vi "count_clients_recursively_VCTP.vi"(7 "Nested type desc.":cluster{"Type descriptor":u8, "Data":string} {"Type descriptor" items=["Void"=0, "NumberI8"=1, "NumberI16"=2, "NumberI32"=3, "NumberI64"=4, "NumberU8"=5, "NumberU16"=6, "NumberU32"=7, "NumberU64"=8, "NumberSGL"=9, "NumberDBL"=10, "NumberEXT"=11, "NumberCSG"=12, "NumberCDB"=13, "NumberCXT"=14, "UnitI8"=17, "UnitI16"=18, "UnitI32"=19, "UnitI64"=20, "UnitU8"=21, "UnitU16"=22, "UnitU32"=23, "UnitU64"=24, "UnitSGL"=25, "UnitDBL"=26, "UnitEXT"=27, "UnitCSG"=28, "UnitCDB"=29, "UnitCXT"=30, "BoolU16"=32, "Bool"=33, "String"=48, "String2"=49, "Path"=50, "Picture"=51, "CString"=52, "PascalString"=53, "Tag"=55, "SubString"=63, "Array"=64, "ArrayDataPtr"=65, "SubArray"=79, "Cluster"=80, "LVVariant"=83, "MeasureData"=84, "ComplexFixedPt"=94, "FixedPoint"=95, "Block"=96, "TypeBlock"=97, "VoidBlock"=98, "AlignedBlock"=99, "RepeatedBlock"=100, "AlignmntMarker"=101, "Refnum"=112, "Set"=115, "Map"=116, "PointerNumber"=128, "PointerNumberI8"=129, "PointerNumberI16"=130, "PointerNumberI32"=131, "PointerNumberI64"=132, "PointerNumberU8"=133, "PointerNumberU16"=134, "PointerNumberU32"=135, "PointerNumberU64"=136, "PointerNumberSGL"=137, "PointerNumberDBL"=138, "PointerNumberEXT"=139, "PointerNumberCSG"=140, "PointerNumberCDB"=141, "PointerNumberCXT"=142, "ArrayInterfc"=160, "InterfcToData"=161, "Terminal"=240, "TypeDef"=241, "PolyVI"=242]}, 8 "error in (no error)":errorcluster, 9 "Control counts in (0)":T1, 10 "Type descriptor index":i32, 11 "VCTP type descriptor list":refnum<data-value>) -> (0 "error out":errorcluster, 1 "Control counts out":T1, 3 "Type descriptor list dup":refnum<data-value>)   [LabVIEW 2020]
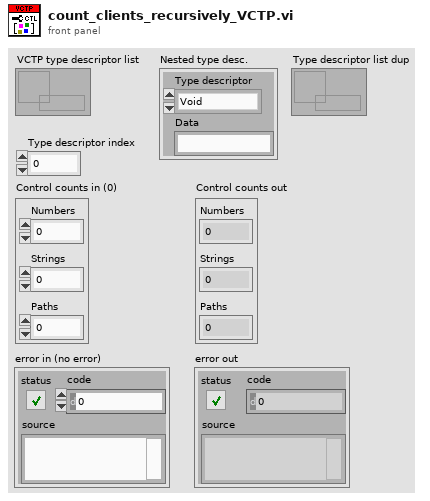
[diagram p1: front panel]
types:
  T1 = cluster{"Numbers":i32, "Strings":i32, "Paths":i32}
  T2 = cluster{"field0":i16, "field2":i16, "field4":i16, "idx":i16}[]
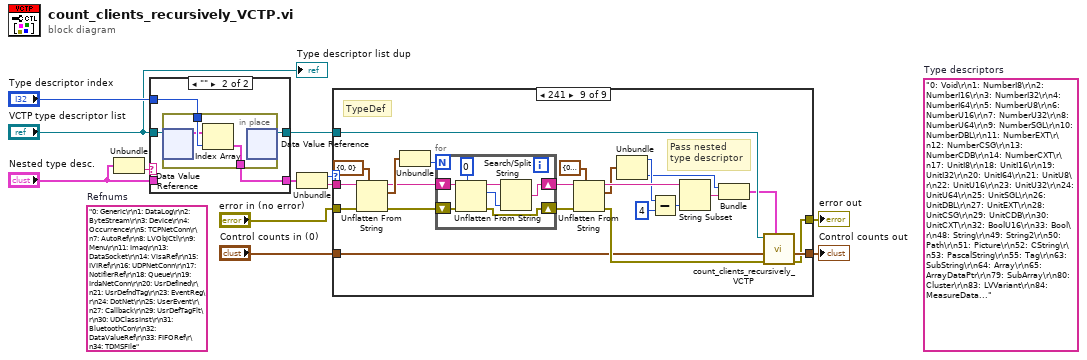
[diagram p0: block diagram]
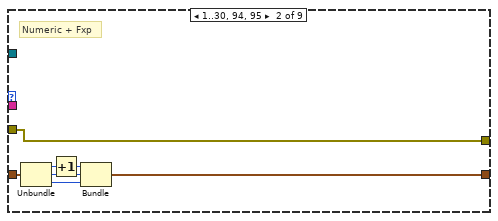
[diagram p4: hidden frame]
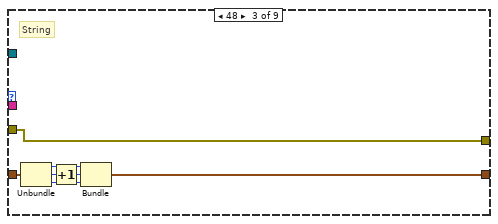
[diagram p5: hidden frame]
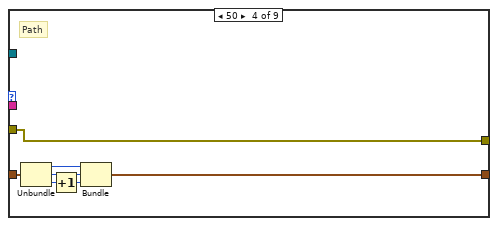
[diagram p6: hidden frame]
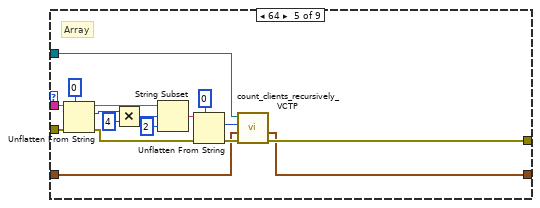
[diagram p7: hidden frame]
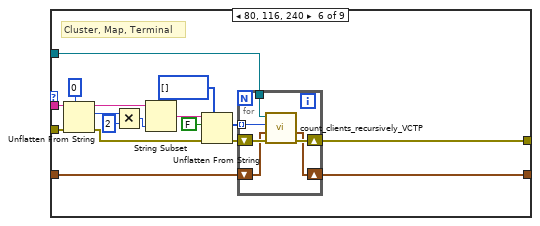
[diagram p8: hidden frame]
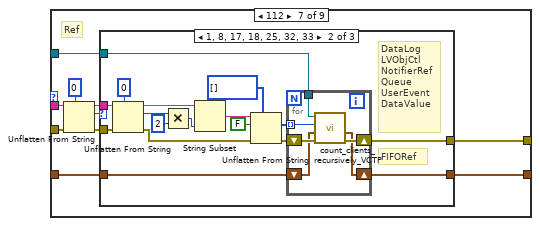
[diagram p9: hidden frame]
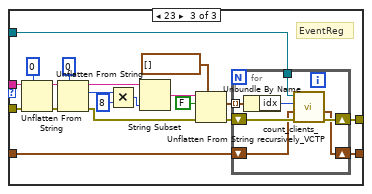
[diagram p11: hidden frame]
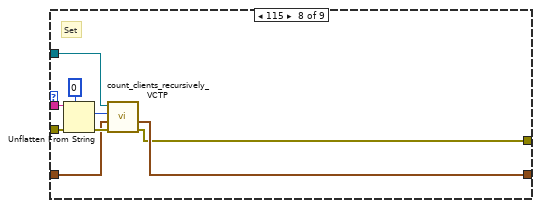
[diagram p12: hidden frame]
diagram:
  (unwired) "0: Generic\r\n1: DataLog\r\n2: ByteStream\r\n3: Device\r\n4: Occurrence\r\n5: TCPNetConn\r\n7: AutoRef\r\n8: LVObjCtl\r\n9: Menu\r\n11: Imaq\r\n13: DataSocket\r\n14: VisaRef\r\n15: IVIRef\r\n16: UDPNetConn\r\n17: NotifierRef\r\n18: Queue\r\n19: IrdaNetConn\r\n20: UsrDefined\r\n21: UsrDefndTag\r\n23: EventReg\r\n24: DotNet\r\n25: UserEvent\r\n27: Callback\r\n29: UsrDefTagFlt\r\n30: UDClassInst\r\n31: BluetoothCon\r\n32: DataValueRef\r\n33: FIFORef\r\n34: TDMSFile"  # Refnums
  (unwired) "0: Void\r\n1: NumberI8\r\n2: NumberI16\r\n3: NumberI32\r\n4: NumberI64\r\n5: NumberU8\r\n6: NumberU16\r\n7: NumberU32\r\n8: NumberU64\r\n9: NumberSGL\r\n10: NumberDBL\r\n11: NumberEXT\r\n12: NumberCSG\r\n13: NumberCDB\r\n14: NumberCXT\r\n17: UnitI8\r\n18: UnitI16\r\n19: UnitI32\r\n20: UnitI64\r\n21: UnitU8\r\n22: UnitU16\r\n23: UnitU32\r\n24: UnitU64\r\n25: UnitSGL\r\n26: UnitDBL\r\n27: UnitEXT\r\n28: UnitCSG\r\n29: UnitCDB\r\n30: UnitCXT\r\n32: BoolU16\r\n33: Bool\r\n48: String\r\n49: String2\r\n50: Path\r\n51: Picture\r\n52: CString\r\n53: PascalString\r\n55: Tag\r\n63: SubString\r\n64: Array\r\n65: ArrayDataPtr\r\n79: SubArray\r\n80: Cluster\r\n83: LVVariant\r\n84: MeasureData\r\n94: ComplexFixedPt\r\n95: FixedPoint\r\n96: Block\r\n97: TypeBlock\r\n98: VoidBlock\r\n99: AlignedBlock\r\n100: RepeatedBlock\r\n101: AlignmntMarker\r\n112: Refnum\r\n115: Set\r\n116: Map\r\n128: PointerNumber\r\n129: PointerNumberI8\r\n130: PointerNumberI16\r\n131: PointerNumberI32\r\n132: PointerNumberI64\r\n133: PointerNumberU8\r\n134: PointerNumberU16\r\n135: PointerNumberU32\r\n136: PointerNumberU64\r\n137: PointerNumberSGL\r\n138: PointerNumberDBL\r\n139: PointerNumberEXT\r\n140: PointerNumberCSG\r\n141: PointerNumberCDB\r\n142: PointerNumberCXT\r\n160: ArrayInterfc\r\n161: InterfcToData\r\n240: Terminal\r\n241: TypeDef\r\n242: PolyVI"  # Type descriptors
  n1 = Unbundle("Nested type desc.") -> ("Data"=w3:string)  [unwired: 1 out]
  n2 = case shown="\"\"" w3 {
    tunnel: "VCTP type descriptor list" -> [w14 w18]
    tunnel: "Type descriptor index" -> [_ w17]
    tunnel: [w13 w16] -> w11
    tunnel: [w14 w15] -> w6
    tunnel: "Nested type desc." -> [w13 _]
    frame Default {
    }
    frame "" {
      n3 = in-place {
        in-place-border: w17 -> [w21]
        in-place-border: [w19] -> w16
        n4 = in-place-dvr #1(w18) -> (w20:cluster{"Type descriptor":u8, "Data":string}[])  [unwired: 1 out]
        n5 = Index Array(array=w20, index=w21) -> (element=w19:cluster{"Type descriptor":u8, "Data":string})
        n6 = in-place-dvr #1() -> (w15:refnum<data-value>)  [unwired: 1 in, 1 out]
      }
    }
  }
  n7 = Unbundle(w11) -> ("Type descriptor"=w10:u8, "Data"=w8:string)
  n8 = case shown="241" w10 {
    tunnel: "error in (no error)" -> [w22 w24 w31 w38 w57 w66 w92 w153 w165]
    tunnel: [w23 w25 w35 w43 w45 w62 w86 w148 w159] -> w5
    tunnel: [w22 w24 w31 w38 w46 w63 w85 w147 w158] -> w4
    tunnel: "Control counts in (0)" -> [w23 w30 w37 w44 w47 w65 w87 w149 w160]
    tunnel: w8 -> [_ _ _ _ w58 w67 w94 w155 w164]
    tunnel: w6 -> [_ _ _ _ w50 w64 w88 w152 w157]
    frame Default {
    }
    frame 1..30, 94, 95 {
      # "Numeric + Fxp"
      n9 = Unbundle(w30) -> ("Numbers"=w29:i32, "Strings"=w27:i32, "Paths"=w26:i32)
      n10 = Increment(x=w29) -> (x+1=w28:i32)
      n11 = Bundle(w28, "Strings"=w27, "Paths"=w26) -> (w25:cluster{i32, "Strings":i32, "Paths":i32})  [unwired: 1 in]
    }
    frame 48 {
      # "String"
      n12 = Unbundle(w37) -> ("Numbers"=w34:i32, "Strings"=w33:i32, "Paths"=w36:i32)
      n13 = Increment(x=w33) -> (x+1=w32:i32)
      n14 = Bundle("Numbers"=w34, w32, "Paths"=w36) -> (w35:cluster{"Numbers":i32, i32, "Paths":i32})  [unwired: 1 in]
    }
    frame 50 {
      # "Path"
      n15 = Unbundle(w44) -> ("Numbers"=w42:i32, "Strings"=w40:i32, "Paths"=w41:i32)
      n16 = Increment(x=w41) -> (x+1=w39:i32)
      n17 = Bundle("Numbers"=w42, "Strings"=w40, w39) -> (w43:cluster{"Numbers":i32, "Strings":i32, i32})  [unwired: 1 in]
    }
    frame 64 {
      # "Array"
      n18 = Unflatten From String(type=i16 0, binary string=w58, error in (no error)=w57) -> (rest of the binary string=w56:string, value=w60:i16, error out=w51:errorcluster)  [unwired: 2 in]
      n19 = Multiply(x=w60, y=i16 4) -> (x*y=w55:i16)
      n20 = String Subset(string=w56, offset (0)=w55, length (rest)=2 ("length (rest)")) -> (substring=w52:string)
      n21 = Unflatten From String(type=i16 0, binary string=w52, error in (no error)=w51) -> (value=w49:i16, error out=w48:errorcluster)  [unwired: 2 in, 1 out]
      n22 = call "count_clients_recursively_VCTP.vi"("error in (no error)"=w48, "Control counts in (0)"=w47, "Type descriptor index"=w49, "VCTP type descriptor list"=w50) -> ("error out"=w46:errorcluster, "Control counts out"=w45:T1)  [unwired: 5 in, 1 out]
    }
    frame 80, 116, 240 {
      # "Cluster, Map, Terminal"
      n23 = Unflatten From String(type=i16 0, binary string=w67, error in (no error)=w66) -> (rest of the binary string=w76:string, value=w71:i16, error out=w72:errorcluster)  [unwired: 2 in]
      n24 = Multiply(x=w71, y=i16 2) -> (x*y=w77:i16)
      n25 = String Subset(string=w76, length (rest)=w77) -> (substring=w78:string)  [unwired: 1 in]
      n26 = Unflatten From String(type=i16[] [] ("index"), binary string=w78, data includes array or string size? (T)=FALSE, error in (no error)=w72) -> (value=w74:i16[], error out=w75:errorcluster)  [unwired: 1 in, 1 out]
      n27 = for {
        tunnel: w74 -> [w83] mode=indexing
        tunnel: w64 -> [w84]
        shift-right: [w81] -> w63
        shift-left: w75 -> [w82]
        shift-right: [w79] -> w62
        shift-left: w65 -> [w80]
        n28 = call "count_clients_recursively_VCTP.vi"("error in (no error)"=w82, "Control counts in (0)"=w80, "Type descriptor index"=w83, "VCTP type descriptor list"=w84) -> ("error out"=w81:errorcluster, "Control counts out"=w79:T1)  [unwired: 5 in, 1 out]
      }
    }
    frame 112 {
      # "Ref"
      n29 = Unflatten From String(type=i16 0, binary string=w94, error in (no error)=w92) -> (rest of the binary string=w91:string, value=w90:i16, error out=w89:errorcluster)  [unwired: 2 in]
      n30 = case shown="1, 8, 17, 18, 25, 32, 33" w90 {
        tunnel: w91 -> [_ w112 w124]
        tunnel: w89 -> [w96 w111 w123]
        tunnel: w88 -> [_ w104 w133]
        tunnel: w87 -> [w95 w102 w131]
        tunnel: [w95 w101 w130] -> w86
        tunnel: [w96 w100 w129] -> w85
        frame Default {
        }
        frame 1, 8, 17, 18, 25, 32, 33 {
          # "FIFORef"
          # "DataLog\nLVObjCtl\nNotifierRef\nQueue\nUserEvent\nDataValue"
          n31 = Unflatten From String(type=i16 0, binary string=w112, error in (no error)=w111) -> (rest of the binary string=w99:string, value=w108:i16, error out=w107:errorcluster)  [unwired: 2 in]
          n32 = Multiply(x=w108, y=i16 2) -> (x*y=w98:i16)
          n33 = String Subset(string=w99, length (rest)=w98) -> (substring=w97:string)  [unwired: 1 in]
          n34 = Unflatten From String(type=i16[] [] ("index"), binary string=w97, data includes array or string size? (T)=FALSE, error in (no error)=w107) -> (value=w105:i16[], error out=w103:errorcluster)  [unwired: 1 in, 1 out]
          n35 = for {
            tunnel: w105 -> [w118] mode=indexing
            tunnel: w104 -> [w119]
            shift-right: [w116] -> w100
            shift-left: w103 -> [w117]
            shift-right: [w114] -> w101
            shift-left: w102 -> [w115]
            n36 = call "count_clients_recursively_VCTP.vi"("error in (no error)"=w117, "Control counts in (0)"=w115, "Type descriptor index"=w118, "VCTP type descriptor list"=w119) -> ("error out"=w116:errorcluster, "Control counts out"=w114:T1)  [unwired: 5 in, 1 out]
          }
        }
        frame 23 {
          # "EventReg"
          n37 = Unflatten From String(type=i16 0, binary string=w124, error in (no error)=w123) -> (rest of the binary string=w122:string, error out=w121:errorcluster)  [unwired: 2 in, 1 out]
          n38 = Unflatten From String(type=i16 0, binary string=w122, error in (no error)=w121) -> (rest of the binary string=w128:string, value=w136:i16, error out=w135:errorcluster)  [unwired: 2 in]
          n39 = Multiply(x=w136, y=i16 8) -> (x*y=w127:i16)
          n40 = String Subset(string=w128, length (rest)=w127) -> (substring=w126:string)  [unwired: 1 in]
          n41 = Unflatten From String(type=T2 [], binary string=w126, data includes array or string size? (T)=FALSE, error in (no error)=w135) -> (value=w134:T2, error out=w132:errorcluster)  [unwired: 1 in, 1 out]
          n42 = for {
            tunnel: w134 -> [w141] mode=indexing
            tunnel: w133 -> [w146]
            shift-right: [w144] -> w129
            shift-left: w132 -> [w145]
            shift-right: [w142] -> w130
            shift-left: w131 -> [w143]
            n43 = Unbundle By Name(w141) -> ("idx"=w140:i16)
            n44 = call "count_clients_recursively_VCTP.vi"("error in (no error)"=w145, "Control counts in (0)"=w143, "Type descriptor index"=w140, "VCTP type descriptor list"=w146) -> ("error out"=w144:errorcluster, "Control counts out"=w142:T1)  [unwired: 5 in, 1 out]
          }
        }
      }
    }
    frame 115 {
      # "Set"
      n45 = Unflatten From String(type=i16 0, binary string=w155, error in (no error)=w153) -> (value=w151:i16, error out=w150:errorcluster)  [unwired: 2 in, 1 out]
      n46 = call "count_clients_recursively_VCTP.vi"("error in (no error)"=w150, "Control counts in (0)"=w149, "Type descriptor index"=w151, "VCTP type descriptor list"=w152) -> ("error out"=w147:errorcluster, "Control counts out"=w148:T1)  [unwired: 5 in, 1 out]
    }
    frame 241 {
      # "Pass nested\ntype descriptor"
      # "TypeDef"
      n47 = Unflatten From String(type=cluster{"Flags":i32, "NumStr":i32} {"Flags"=0, "NumStr"=0}, binary string=w164, error in (no error)=w165) -> (rest of the binary string=w166:string, value=w177:cluster{"Flags":i32, "NumStr":i32}, error out=w167:errorcluster)  [unwired: 2 in]
      n48 = Unbundle(w177) -> ("NumStr"=w178:i32)  [unwired: 1 out]
      n49 = for {
        N: w178 -> [_]
        shift-right: [w180] -> w171
        shift-left: w166 -> [w184]
        shift-right: [w179] -> w173
        shift-left: w167 -> [w183]
        n50 = Unflatten From String(type=u8 0, binary string=w184, error in (no error)=w183) -> (rest of the binary string=w182:string, value=w181:u8, error out=w179:errorcluster)  [unwired: 2 in]
        n51 = Search/Split String(string=w182, offset (0)=w181) -> (match + rest of string=w180:string)  [unwired: 1 in, 2 out]
      }
      n52 = Unflatten From String(type=cluster{"length":i16, "flags":u8, "type":u8} {"length"=0, "flags"=0, "type"=0}, binary string=w171, error in (no error)=w173) -> (rest of the binary string=w175:string, value=w169:cluster{"length":i16, "flags":u8, "type":u8}, error out=w161:errorcluster)  [unwired: 2 in]
      n53 = Unbundle(w169) -> ("length"=w170:i16, "type"=w162:u8)  [unwired: 1 out]
      n54 = Subtract(x=w170, y=i16 4) -> (x-y=w174:i16)
      n55 = String Subset(string=w175, length (rest)=w174) -> (substring=w163:string)  [unwired: 1 in]
      n56 = Bundle("type"=w162, w163) -> (w156:cluster{"type":u8, string})  [unwired: 1 in]
      n57 = call "count_clients_recursively_VCTP.vi"("Nested type desc."=w156, "error in (no error)"=w161, "Control counts in (0)"=w160, "VCTP type descriptor list"=w157) -> ("error out"=w158:errorcluster, "Control counts out"=w159:T1)  [unwired: 5 in, 1 out]
    }
  }
  "error out" <- w4
  "Control counts out" <- w5
  "Type descriptor list dup" <- "VCTP type descriptor list"
